vi "mining.vi"(7 "httpRequestID":u32) -> ()   [LabVIEW 2011]
doc: "This VI is a state machine that can be ran from a Browser."
uses:
  server/database/Users/User Record.ctl
  <vilib>/wsapi/NI_WebServices.lvlib
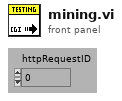
[diagram p1: front panel]
types:
  T1 = typedef "User Record.ctl" = cluster{"ixUser":i32, "sxUsername":string, "sLastName":string, "sFirstName":string, "sEmail":string, "sPassword":string, "tLoginTime":timestamp, "sLoginComputer":string, "fAdministrator":bool, "fRunSequences":bool, "fModifySequences":bool, "fRunScenarios":bool, "fModifyScenarios":bool, "fModifyTemplates":bool, "fModifyUsers":bool, "fModifyStations":bool, "fModifyFields":bool}
  T2 = typedef "Connection Refnum.ctl" = cluster{"Environment Handle":i32, "Connection Handle":i32}
  T3 = typedef "Keyed Array.ctl" = cluster{"keys":string[], "values":string[]}
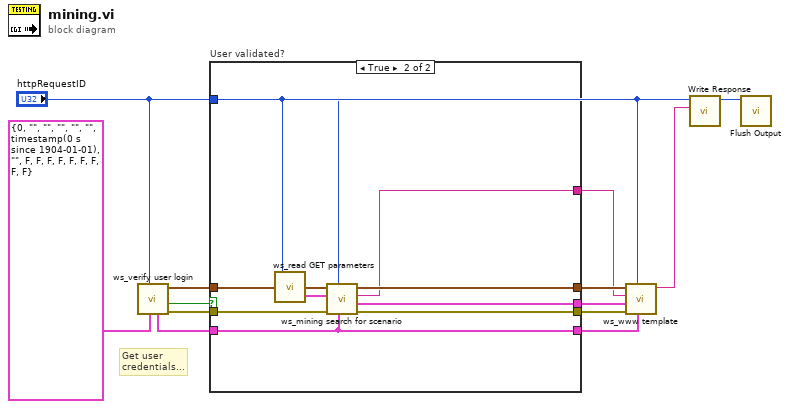
[diagram p0: block diagram]
diagram:
  # "Get user \ncredentials..."
  n1 = call "ws_verify user login.vi"("Required Permisions"=T1 {"ixUser"=0, "sxUsername"="", "sLastName"="", "sFirstName"="", "sEmail"="", "sPassword"="", "tLoginTime"=timestamp(0 s since 1904-01-01), "sLoginComputer"="", "fAdministrator"=FALSE, "fRunSequences"=FALSE, "fModifySequences"=FALSE, "fRunScenarios"=FALSE, "fModifyScenarios"=FALSE, "fModifyTemplates"=FALSE, "fModifyUsers"=FALSE, "fModifyStations"=FALSE, "fModifyFields"=FALSE} ("User Record"), "httpRequestID"="httpRequestID") -> ("error out"=w13:errorcluster, "User Verified\nand Spartan\nAuthorized?"=w12:bool, "DB Connection Ref"=w11:T2, "User"=w10:T1)  [unwired: 6 in]
  n2 = case "User validated?" shown="True" w12 {
    tunnel: w10 -> [w14 w19]
    tunnel: w11 -> [w15 w24]
    tunnel: w13 -> [w16 w23]
    tunnel: [w16 w22] -> w7
    tunnel: [w15 w25] -> w8
    tunnel: [_ w20] -> w1
    tunnel: [_ w21] -> w6
    tunnel: [w14 w19] -> w5
    tunnel: "httpRequestID" -> [_ w17]
    frame False {
    }
    frame True {
      n3 = call "ws_read GET parameters.vi"("httpRequestID"=w17) -> ("GET query params"=w18:T3)  [unwired: 2 in]
      n4 = call "ws_mining search for scenario.vi"("User"=w19, "httpRequestID"=w17, "error in (no error)"=w23, "GET (empty)"=w18, "Connection Refnum"=w24) -> ("error out"=w22:errorcluster, "Template Keys"=w21:T3, "Template"=w20:string, "Connection Refnum"=w25:T2)  [unwired: 3 in]
    }
  }
  n5 = call "ws_www template.vi"("User"=w5, "httpRequestID"="httpRequestID", "error in (no error)"=w7, "Template Keys (empty)"=w6, "Template (\"\")"=w1, "DB Connection Ref"=w8) -> ("HTTP Template Content"=w3:string)  [unwired: 5 in]
  n6 = call <vilib>:"Write Response.vi"("response string"=w3, "httpRequestID"="httpRequestID") -> ("httpRequestID out"=w2:u32)  [unwired: 8 in, 1 out]
  n7 = call <vilib>:"Flush Output.vi"("httpRequestID"=w2) -> ()  [unwired: 9 in, 2 out]
